vi "Data Logger.vi"() -> ()   [LabVIEW 2020]
uses:
  epl-vi-lib/Utility VIs/Buttons/KCheckmarkBoolean 2.ctl
  Typedefs/DL-Channel Spec.ctl
  <vilib>/DAQmx/read.llb/DAQmx Read (Analog 1D Wfm NChan NSamp).vi
  Typedefs/DL-Globals.vi
  <vilib>/DAQmx/miscellaneous.llb/DAQmx Fill In Error Info.vi
  <vilib>/sound2/lvsound2.llb/Sound File Write (DBL).vi
  <resource>/objmgr/daqmx.rc
panel:
  in  "Trigger":enum16{"Internal", "External"}(ring)
  in  ".wav file":T1 caption="Save as .wav file"
  in  "Duration (s)":dbl=1.0 min=1.0
  in  "Device":u16(ring) items=["PXI1Slot4"]
  in  "Filestem":string
  in  "Folder":path
  in  "Sampling rate (Hz)":dbl=1000.0 min=1000.0 max=200000.0
  in  "AI":T2
  out "Filename":string
  out "finished":errorcluster
  out "Graph":dbl[][](graph)
  in  "Start":bool
  in  "Stop":bool
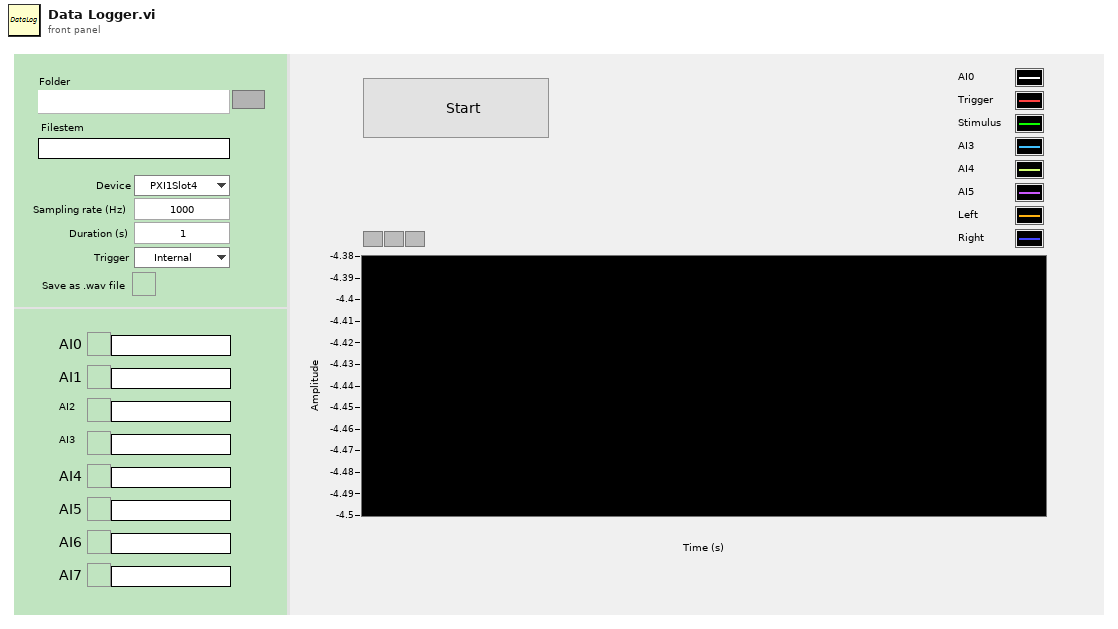
[diagram p1: front panel]
types:
  T1 = typedef "KCheckmarkBoolean 2.ctl" = bool
  T2 = cluster{"Ch0":cluster{"active":T1, "name":string}, "Ch1":cluster{"active":T1, "name":string}, "Ch2":cluster{"active":T1, "name":string}, "Ch3":cluster{"active":T1, "name":string}, "Ch4":cluster{"active":T1, "name":string}, "Ch5":cluster{"active":T1, "name":string}, "Ch6":cluster{"active":T1, "name":string}, "Ch7":cluster{"active":T1, "name":string}}
  T3 = typedef "DL-IPC.ctl" = cluster{"Acquire":refnum<queue>, "Analysis":refnum<queue>, "Data":refnum<queue>}
  T4 = typedef "DL-Channel Spec.ctl" = cluster{"active":bool, "name":string}
  T5 = enum8{"Enabled", "Disabled", "Disabled and Grayed Out"}
  T6 = typedef "DL-Configuration.ctl" = cluster{"Folder":path, "Filestem":string, "Device":string, "Fs (Hz)":dbl, "T (s)":dbl, "AI":T4[], "frame size (s)":dbl, ".wav file":bool, "Trigger":enum16{"Internal", "External"}, "remote":bool}
  T7 = typedef "Sound File Refnum.ctl" = refnum<file>
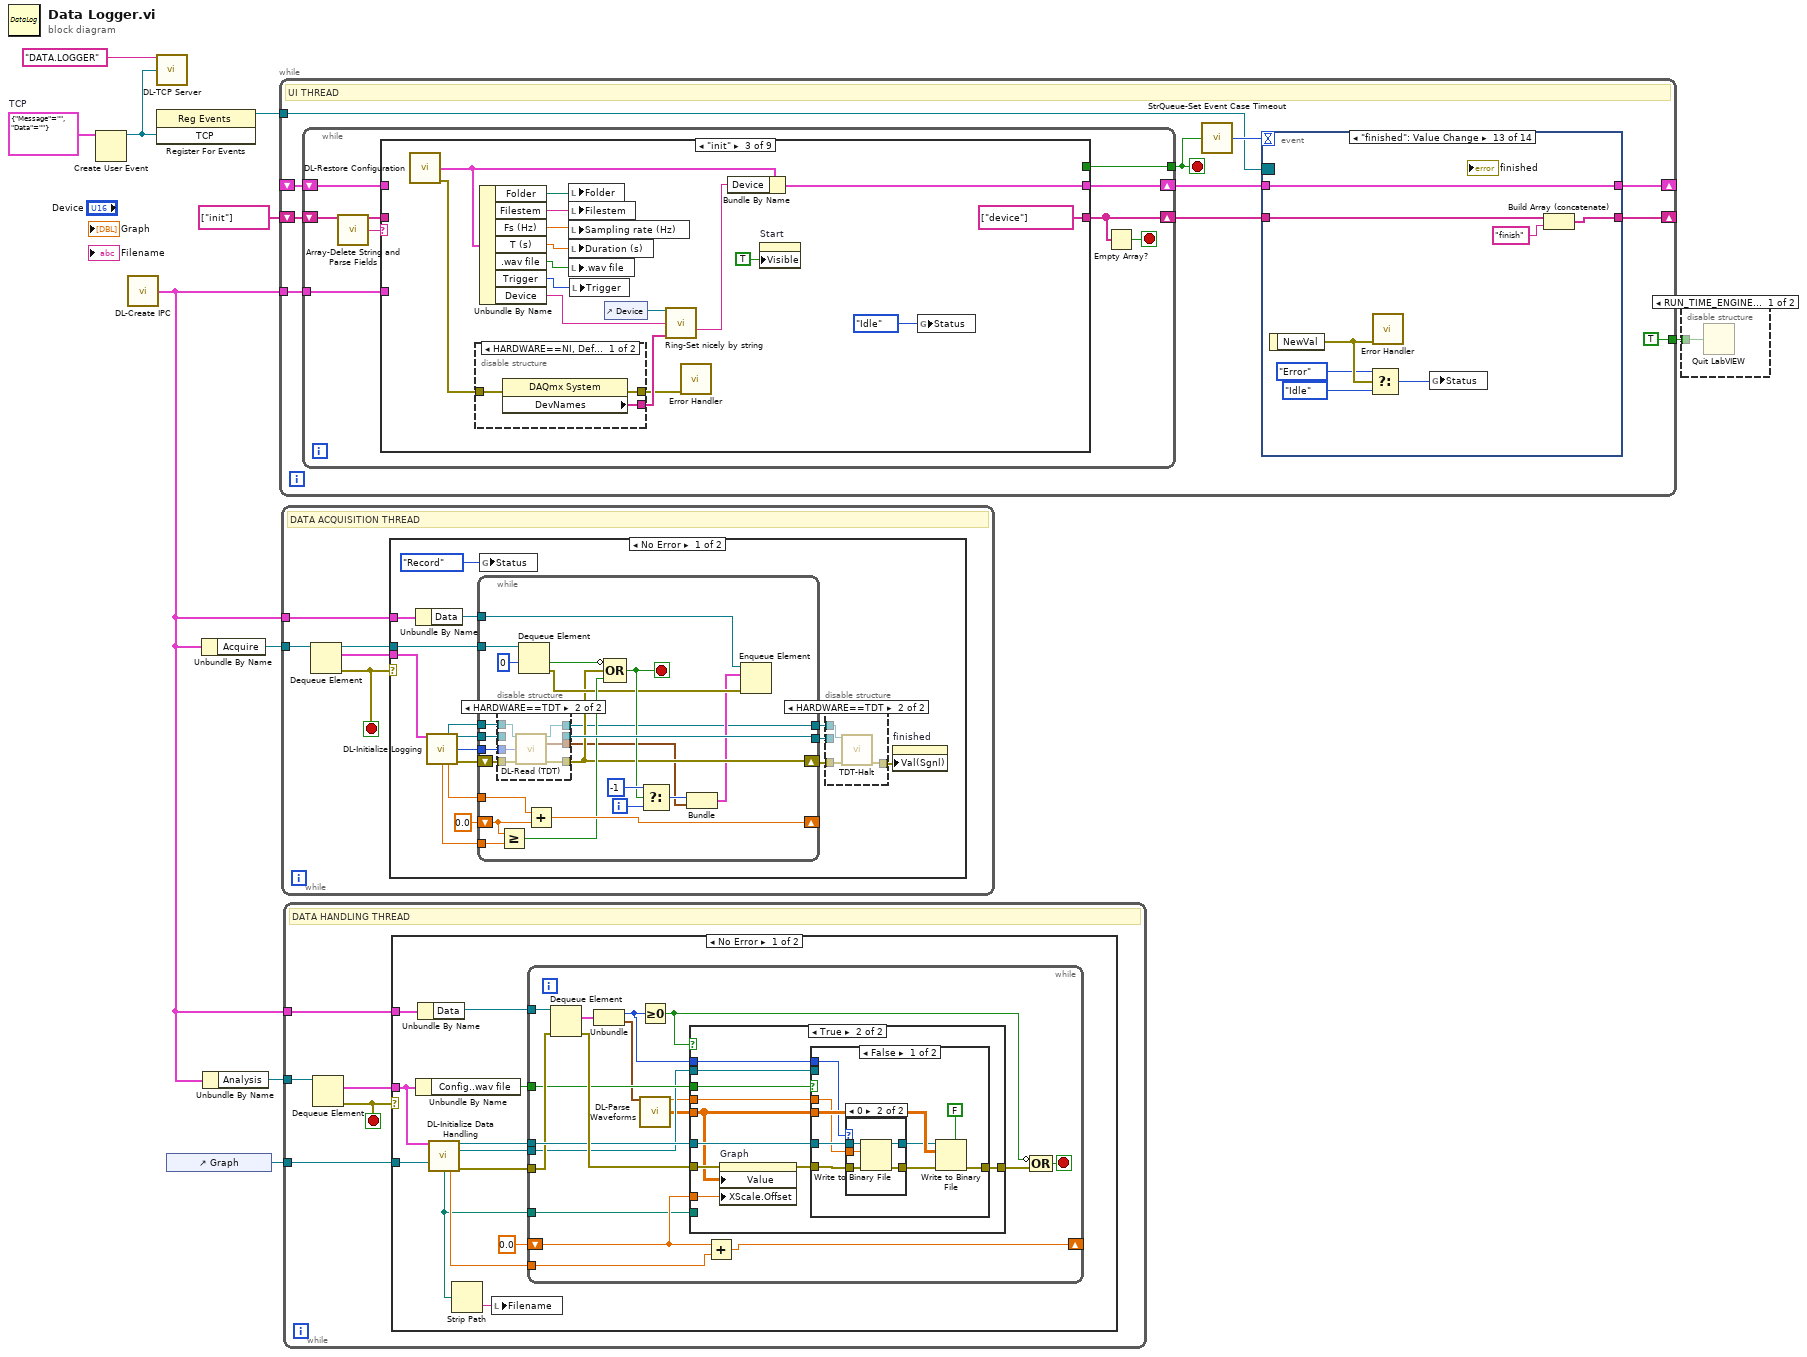
[diagram p0: block diagram]
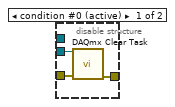
[diagram p2: hidden frame]
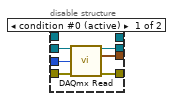
[diagram p3: hidden frame]
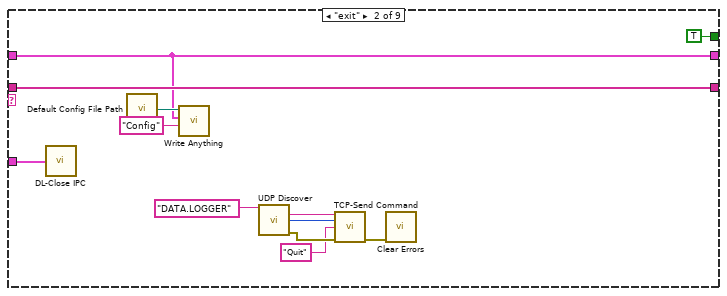
[diagram p6: hidden frame]
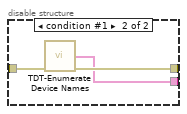
[diagram p7: hidden frame]
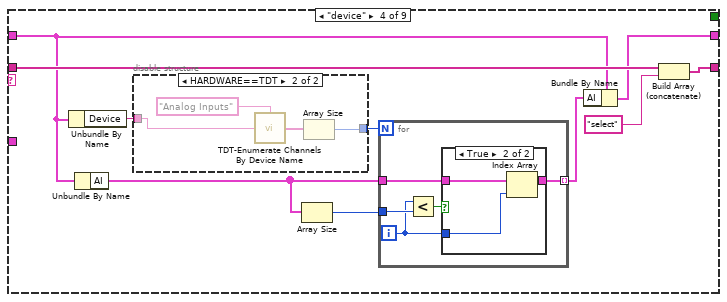
[diagram p8: hidden frame]
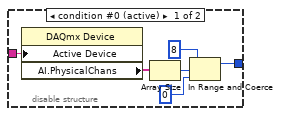
[diagram p9: hidden frame]
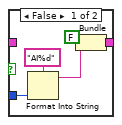
[diagram p10: hidden frame]
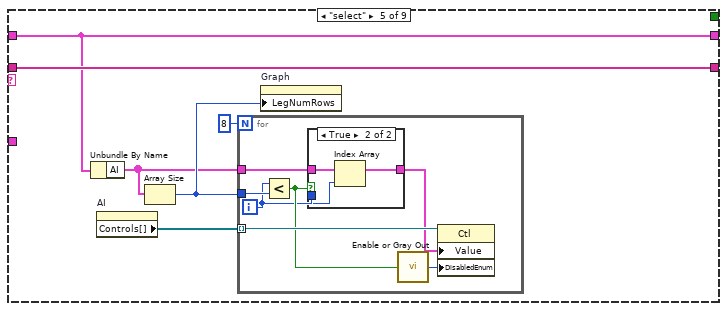
[diagram p11: hidden frame]
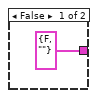
[diagram p12: hidden frame]
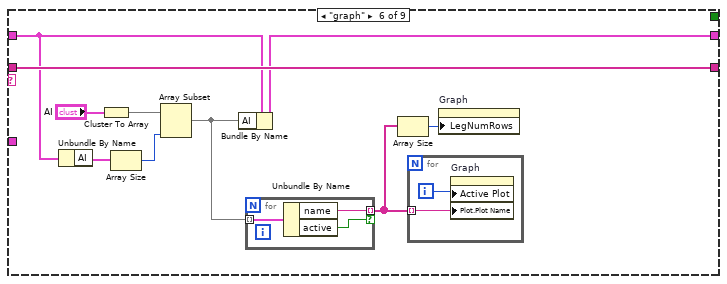
[diagram p13: hidden frame]
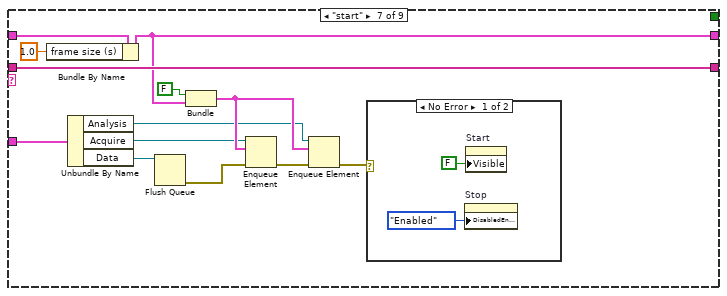
[diagram p14: hidden frame]
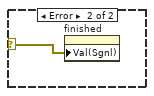
[diagram p15: hidden frame]
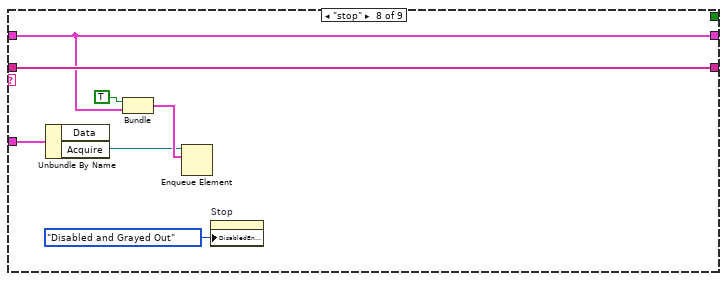
[diagram p16: hidden frame]
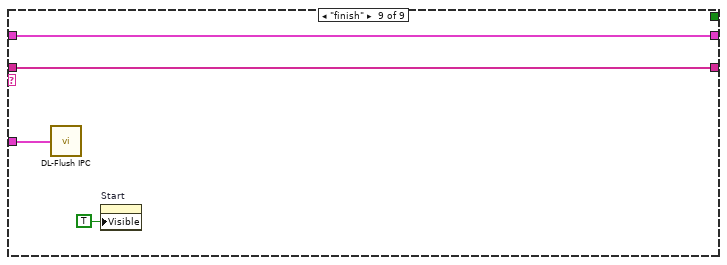
[diagram p17: hidden frame]
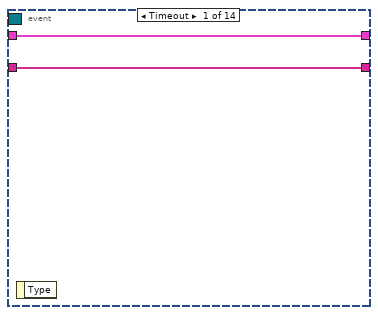
[diagram p18: hidden frame]
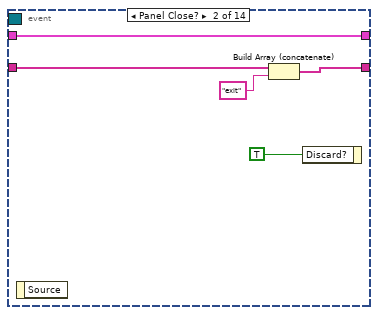
[diagram p19: hidden frame]
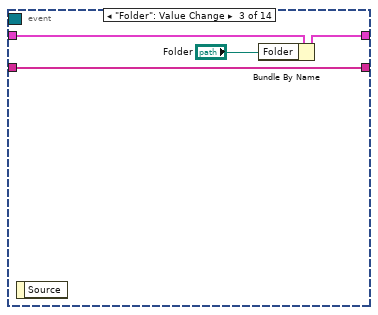
[diagram p20: hidden frame]
diagram:
  w1 = cluster{"Message":string, "Data":string} {"Message"="", "Data"=""}  # TCP
  n1 = Create User Event(user event datatype=w1) -> (user event=w2:refnum<user-event>)  [unwired: 1 in, 1 out]
  n2 = call "DL-Create IPC.vi"() -> ("IPC"=w8:T3)  [unwired: 15 in]
  n3 = call "DL-TCP Server.vi"("callsign"="DATA.LOGGER", "TCP Event"=w2) -> ()  [unwired: 14 in]
  n4 = register-events(w2) -> (reference out=w3:refnum<event-registration>)  [unwired: 2 in, 1 out]
  n5 = control-ref of="Graph"() -> (w7:refnum<vi>)
  n6 = Unbundle By Name(w8) -> ("Acquire"=w10:refnum<queue>)
  n7 = Unbundle By Name(w8) -> ("Analysis"=w9:refnum<queue>)
  n8 = while {
    shift-right: [w19] -> _
    shift-left: _ -> [w18]
    tunnel: w8 -> [w21]
    tunnel: [TRUE] -> w6
    shift-right: [w16] -> _
    shift-left: string[] ["init"] -> [w12]
    tunnel: w3 -> [w11]
    stop <- w13 stop-if-true
    # "UI THREAD"
    n9 = while {
      shift-right: [w30] -> w17
      shift-left: w12 -> [w27]
      tunnel: [w28] -> w13
      tunnel: w21 -> [w24]
      shift-right: [w23] -> w20
      shift-left: w18 -> [w22]
      stop <- w29 stop-if-true
      n10 = call "Array-Delete String and Parse Fields.vi"("Array in"=w27) -> ("Array out"=w26:string[], "Field 1"=w25:string)  [unwired: 10 in, 3 out]
      n11 = case shown="\"init\"" w25 {
        tunnel: w26 -> [w32 w44 _ w77 w106 w127 w145 w155 w159]
        tunnel: [w32 w44 string[] ["device"] ("Array out") w69 w106 w127 w145 w155 w159] -> w30
        tunnel: [_ TRUE _ _ _ _ _ _ _] -> w28
        tunnel: w24 -> [_ w43 _ _ _ _ w136 w151 w157]
        tunnel: [w31 w39 w50 w70 w101 w118 w134 w150 w158] -> w23
        tunnel: w22 -> [w31 w39 _ w71 w101 w119 w135 w150 w158]
        frame Default {
        }
        frame "exit" {
          n12 = call "DL-Close IPC.vi"("IPC"=w43) -> ()  [unwired: 14 in, 1 out]
          n13 = call "Default Config File Path.vi"() -> ("Default config file name"=w41:path)
          n14 = call "Write Anything.vi"("Section Name (Name of \"Anything\")"="Config" ("Section Name (Name of \"Anything\")"), "Anything"=w39, "Path (dialog)"=w41) -> ()  [unwired: 7 in, 2 out]
          n15 = call "UDP Discover.vi"("Name"="DATA.LOGGER" ("callsign")) -> ("Address"=w38:string, "Port"=w37:i32, "error out"=w36:errorcluster)  [unwired: 10 in, 2 out]
          n16 = call "TCP-Send Command.vi"("PXI Address"=w38, "Port"=w37, "Command"="Quit", "error in (no error)"=w36) -> ("error out"=w33:errorcluster)  [unwired: 11 in]
          n17 = call <vilib>:"Clear Errors.vi"("error in (no error)"=w33) -> ()  [unwired: 5 in, 2 out]
        }
        frame "init" {
          n18 = call "DL-Restore Configuration.vi"() -> ("Config"=w51:T6, "error out"=w48:errorcluster)  [unwired: 14 in]
          n19 = disable-structure shown="HARDWARE==NI, Default" {
            disable-tunnel: w48 -> [w63 w67]
            disable-tunnel: [w62 w65] -> w47
            disable-tunnel: [w64 w66] -> w46
            frame condition #0 (active) {
              n20 = property class="DAQmx System"(error in=w63) -> (error out=w64:errorcluster, "DevNames"=w62:tag[])  [unwired: 1 in, 1 out]
            }
            frame condition #1 {
              n21 = call "TDT-Enumerate Device Names.vi"("error in (no error)"=w67) -> ("Device names"=w65:string[], "error out"=w66:errorcluster)  [unwired: 13 in]
            }
          }
          n22 = Unbundle By Name(w51) -> ("Folder"=w52:path, "Filestem"=w53:string, "Fs (Hz)"=w54:dbl, "T (s)"=w57:dbl, ".wav file"=w59:bool, "Trigger"=w60:enum16{"Internal", "External"}, "Device"=w56:string)
          n23 = local write "Folder"(w52) -> ()
          n24 = local write "Filestem"(w53) -> ()
          n25 = local write "Sampling rate (Hz)"(w54) -> ()
          n26 = local write "Duration (s)"(w57) -> ()
          n27 = local write ".wav file"(w59) -> ()
          n28 = local write "Trigger"(w60) -> ()
          n29 = control-ref of="Device"() -> (w55:refnum<vi>)
          n30 = call "Ring-Set nicely by string.vi"("Ring in"=w55, "Device"=w56, "Strings []"=w47) -> ("Selection"=w61:string)  [unwired: 8 in, 4 out]
          n31 = call "Error Handler.vi"("error in (no error)"=w46) -> ()  [unwired: 12 in, 3 out]
          n32 = Bundle By Name(cluster=w51, "Device"=w61) -> (w50:T6)
          n33 = property on="Start" class="Bool"("Visible"=TRUE) -> ()  [unwired: 2 in, 2 out]
          n34 = global write "DL-Globals.vi" "Status"(enum16{"Idle", "Record", "Error"}."Idle" ("Status")) -> ()
        }
        frame "device" {
          n35 = Unbundle By Name(w71) -> ("Device"=w72:string)
          n36 = Unbundle By Name(w71) -> ("AI"=w73:T4[])
          n37 = disable-structure shown="HARDWARE==TDT" {
            disable-tunnel: [w83 w85] -> w76
            disable-tunnel: w72 -> [w80 w87]
            frame condition #0 (active) {
              n38 = property class="DAQmx Device"("Active Device"=w80) -> ("AI.PhysicalChans"=w81:tag[])  [unwired: 2 in, 2 out]
              n39 = Array Size(array=w81) -> (size(s)=w82:i32)
              n40 = In Range and Coerce(upper limit=8, x=w82, lower limit=0) -> (coerced(x)=w83:i32)  [unwired: 1 out]
            }
            frame condition #1 {
              n41 = call "TDT-Enumerate Channels By Device Name.vi"("Type"="Analog Inputs", "Device"=w87) -> ("IO Channels"=w86:string[])  [unwired: 13 in]
              n42 = Array Size(array=w86) -> (size(s)=w85:i32)
            }
          }
          n43 = Array Size(array=w73) -> (size(s)=w74:i32)
          n44 = for {
            N: w76 -> [_]
            tunnel: w73 -> [w91]
            tunnel: w74 -> [w92]
            tunnel: [w89] -> w75 mode=indexing
            i -> [w88]
            n45 = Less?(x=w88, y=w92) -> (x < y?=w90:bool)
            n46 = case shown="True" w90 {
              tunnel: w91 -> [_ w100]
              tunnel: [w96 w99] -> w89
              tunnel: w88 -> [w97 w98]
              frame False {
                n47 = Format Into String(format string="AI%d", w97) -> (resulting string=w93:string)  [unwired: 2 in, 1 out]
                n48 = Bundle(FALSE, w93) -> (w96:cluster{bool, string})  [unwired: 1 in]
              }
              frame True {
                n49 = Index Array(array=w100, index=w98) -> (element=w99:T4)
              }
            }
          }
          n50 = Bundle By Name(cluster=w71, "AI"=w75) -> (w70:T6)
          n51 = Build Array (concatenate)(w77, "select") -> (w69:string[])
        }
        frame "select" {
          n52 = Unbundle By Name(w101) -> ("AI"=w103:T4[])
          n53 = property on="AI" class="Clust (strict)"() -> ("Controls[]"=w104:refnum<vi>[])  [unwired: 2 in, 2 out]
          n54 = Array Size(array=w103) -> (size(s)=w105:i32)
          n55 = for {
            N: 8 -> [_]
            tunnel: w103 -> [w111]
            tunnel: w105 -> [w113]
            tunnel: w104 -> [w112] mode=indexing
            i -> [w107]
            n56 = Less?(x=w107, y=w113) -> (x < y?=w109:bool)
            n57 = case shown="True" w109 {
              tunnel: w111 -> [_ w117]
              tunnel: [T4 {"active"=FALSE, "name"=""} ("Channel") w115] -> w108
              tunnel: w107 -> [_ w116]
              frame False {
              }
              frame True {
                n58 = Index Array(array=w117, index=w116) -> (element=w115:T4)
              }
            }
            n59 = call "Enable or Gray Out.vi"("Boolean"=w109) -> ("Disabled"=w110:T5)
            n60 = property class="Ctl"(reference=w112, "Value"=w108, "DisabledEnum"=w110) -> ()  [unwired: 1 in, 2 out]
          }
          n61 = property on="Graph" class="WFGraph (strict)"("LegNumRows"=w105) -> ()  [unwired: 2 in, 2 out]
        }
        frame "graph" {
          n62 = Unbundle By Name(w119) -> ("AI"=w122:T4[])
          n63 = Cluster To Array(cluster="AI") -> (array=w121:cluster{"active":T1, "name":string}[])
          n64 = Array Size(array=w122) -> (size(s)=w123:i32)
          n65 = Array Subset(array=w121, length=w123) -> (w124:cluster{"active":T1, "name":string}[])  [unwired: 1 in]
          n66 = Bundle By Name(cluster=w119, "AI"=w124) -> (w118:T6)
          n67 = for {
            tunnel: w124 -> [w130] mode=indexing
            tunnel: [w129] -> w126 mode=indexing if=w128
            n68 = Unbundle By Name(w130) -> ("name"=w129:string, "active"=w128:T1)
          }
          n69 = Array Size(array=w126) -> (size(s)=w125:i32)
          n70 = for {
            tunnel: w126 -> [w131] mode=indexing
            i -> [w132]
            n71 = property on="Graph" class="WFGraph (strict)"("Active Plot"=w132, "Plot.Plot Name"=w131) -> ()  [unwired: 2 in, 2 out]
          }
          n72 = property on="Graph" class="WFGraph (strict)"("LegNumRows"=w125) -> ()  [unwired: 2 in, 2 out]
        }
        frame "start" {
          n73 = Bundle By Name(cluster=w135, "frame size (s)"=1.0) -> (w134:T6)
          n74 = Unbundle By Name(w136) -> ("Analysis"=w139:refnum<queue>, "Acquire"=w138:refnum<queue>, "Data"=w143:refnum<queue>)
          n75 = Flush Queue(queue=w143) -> (error out=w144:errorcluster)  [unwired: 1 in, 2 out]
          n76 = Bundle(FALSE, "Config"=w134) -> (w141:cluster{bool, "Config":T6})  [unwired: 1 in]
          n77 = Enqueue Element(queue=w138, element=w141, error in (no error)=w144) -> (error out=w140:errorcluster)  [unwired: 1 in, 2 out]
          n78 = Enqueue Element(queue=w139, element=w141, error in (no error)=w140) -> (error out=w142:errorcluster)  [unwired: 1 in, 2 out]
          n79 = case shown="No Error" w142 {
            selector: w142 -> [_ w148]
            frame No Error {
              n80 = property on="Stop" class="Bool"("DisabledEnum"=T5."Enabled" ("Disabled")) -> ()  [unwired: 2 in, 2 out]
              n81 = property on="Start" class="Bool"("Visible"=FALSE) -> ()  [unwired: 2 in, 2 out]
            }
            frame Error {
              n82 = property on="finished" class="Clust (strict)"("Val(Sgnl)"=w148) -> ()  [unwired: 2 in, 2 out]
            }
          }
        }
        frame "stop" {
          n83 = Unbundle By Name(w151) -> ("Acquire"=w153:refnum<queue>)  [unwired: 1 out]
          n84 = Bundle(TRUE, "Config"=w150) -> (w154:cluster{bool, "Config":T6})  [unwired: 1 in]
          n85 = Enqueue Element(queue=w153, element=w154) -> ()  [unwired: 2 in, 3 out]
          n86 = property on="Stop" class="Bool"("DisabledEnum"=T5."Disabled and Grayed Out" ("Disabled")) -> ()  [unwired: 2 in, 2 out]
        }
        frame "finish" {
          n87 = call "DL-Flush IPC.vi"("IPC"=w157) -> ()  [unwired: 14 in, 1 out]
          n88 = property on="Start" class="Bool"("Visible"=TRUE) -> ()  [unwired: 2 in, 2 out]
        }
      }
      n89 = Empty Array?(array=w30) -> (empty?=w29:bool)
    }
    n90 = call "StrQueue-Set Event Case Timeout.vi"("Quit"=w13) -> ("timeout"=w14:i32)  [unwired: 14 in]
    n91 = event shown="[12] \"finished\": Value Change" {
      selector: w11 -> [_ _ _ _ _ _ _ _ _ _ _ _ _ _]
      dyn-events: _ -> [_ _ _ _ _ _ _ _ _ _ _ _ _ _]
      timeout: w14 -> [_ _ _ _ _ _ _ _ _ _ _ _ _ _]
      tunnel: [w161 w165 w169 w173 w177 w181 w185 w189 w195 w200 w202 w210 w218 w223] -> w19
      tunnel: w20 -> [w161 w165 w170 w174 w178 w182 w186 w190 w196 w200 w206 w210 w218 w225]
      tunnel: w17 -> [w160 w164 w167 w171 w175 w179 w183 w187 w193 w199 w205 w209 w217 w226]
      tunnel: [w160 w163 w167 w171 w175 w179 w183 w187 w192 w198 w204 w208 w216 w220] -> w16
      event Timeout {
        n92 = event-data() -> ()  [unwired: 1 in, 1 out]
      }
      event Panel Close? {
        n93 = event-data() -> ()  [unwired: 1 in, 1 out]
        n94 = Build Array (concatenate)(w164, "exit") -> (w163:string[])
        n95 = event-data("Discard?"=TRUE) -> ()  [unwired: 1 in, 1 out]
      }
      event "Folder": Value Change {
        n96 = event-data() -> ()  [unwired: 1 in, 1 out]
        n97 = Bundle By Name(cluster=w170, "Folder"="Folder") -> (w169:T6)
      }
      event "Filestem": Value Change {
        n98 = event-data() -> ()  [unwired: 1 in, 1 out]
        n99 = Bundle By Name(cluster=w174, "Filestem"="Filestem") -> (w173:T6)
      }
      event "Sampling rate (Hz)": Value Change {
        n100 = event-data() -> ()  [unwired: 1 in, 1 out]
        n101 = Bundle By Name(cluster=w178, "Fs (Hz)"="Sampling rate (Hz)") -> (w177:T6)
      }
      event "Duration (s)": Value Change {
        n102 = event-data() -> ()  [unwired: 1 in, 1 out]
        n103 = Bundle By Name(cluster=w182, "T (s)"="Duration (s)") -> (w181:T6)
      }
      event "Trigger": Value Change {
        n104 = event-data() -> ()  [unwired: 1 in, 1 out]
        n105 = Bundle By Name(cluster=w186, "Trigger"="Trigger") -> (w185:T6)
      }
      event Value Change {
        n106 = event-data() -> ()  [unwired: 1 in, 1 out]
        n107 = Bundle By Name(cluster=w190, ".wav file"=".wav file") -> (w189:T6)
      }
      event "Device": Value Change {
        n108 = event-data() -> ()  [unwired: 1 in, 1 out]
        n109 = property on="Device" class="Ring (strict)"() -> ("RingText.Text"=w194:string)  [unwired: 2 in, 2 out]
        n110 = Bundle By Name(cluster=w196, "Device"=w194) -> (w195:T6)
        n111 = Build Array (concatenate)(w193, "device") -> (w192:string[])
      }
      event "AI": Value Change {
        n112 = event-data() -> ()  [unwired: 1 in, 1 out]
        n113 = Build Array (concatenate)(w199, "graph") -> (w198:string[])
      }
      event "Start": Value Change {
        n114 = event-data() -> ()  [unwired: 1 in, 1 out]
        n115 = Bundle By Name(cluster=w206, "remote"=FALSE) -> (w202:T6)
        n116 = Build Array (concatenate)(w205, "start") -> (w204:string[])
      }
      event "Stop": Value Change {
        n117 = event-data() -> ()  [unwired: 1 in, 1 out]
        n118 = Build Array (concatenate)(w209, "stop") -> (w208:string[])
      }
      event "finished": Value Change {
        n119 = event-data() -> ("NewVal"=w214:errorcluster)  [unwired: 1 in]
        n120 = Select(t=enum16{"Idle", "Record", "Error"}."Error" ("Status"), s=w214, f=enum16{"Idle", "Record", "Error"}."Idle" ("Status")) -> (s? t:f=w211:enum16{"Idle", "Record", "Error"})
        n121 = call "Error Handler.vi"("error in (no error)"=w214) -> ()  [unwired: 12 in, 3 out]
        n122 = global write "DL-Globals.vi" "Status"(w211) -> ()
        n123 = Build Array (concatenate)(w217, "finish") -> (w216:string[])
      }
      event User Event {
        n124 = event-data() -> ("Message"=w224:string, "Data"=w222:string)  [unwired: 1 in]
        n125 = String To Path(string=w222) -> (path=w221:path)
        n126 = case shown="\"Record\"" w224 {
          tunnel: w225 -> [w227 w235 w236]
          tunnel: [w227 w233 w236] -> w223
          tunnel: w221 -> [_ w234 _]
          tunnel: [_ w231 w237] -> w219
          frame Default {
          }
          frame "Record" {
            n127 = Strip Path(path=w234) -> (stripped path=w229:path)  [unwired: 1 out]
            n128 = call <vilib>:"Get File Extension.vi"("file"=w234) -> ("filename without extension"=w230:string)  [unwired: 6 in, 4 out]
            n129 = local write "Folder"(w229) -> ()
            n130 = local write "Filestem"(w230) -> ()
            n131 = Bundle By Name(cluster=w235, "remote"=TRUE, "Folder"=w229, "Filestem"=w230) -> (w233:T6)
            n132 = Build Array("start") -> (w231:string[])
          }
          frame "Stop" {
            n133 = Build Array("stop") -> (w237:string[])
          }
        }
        n134 = Build Array (concatenate)(w226, w219) -> (w220:string[])
      }
    }
  }
  n135 = while {
    tunnel: w10 -> [w243]
    tunnel: w8 -> [w240]
    stop <- w242 stop-if-true
    # "DATA ACQUISITION THREAD"
    n136 = Dequeue Element(queue=w243) -> (queue out=w241:refnum<queue>, element=w239:cluster{"Stop":bool, "Config":T6}, error out=w242:errorcluster)  [unwired: 2 in, 1 out]
    n137 = case shown="No Error" w242 {
      tunnel: w241 -> [w257 _]
      tunnel: w240 -> [w255 _]
      tunnel: w239 -> [w247 _]
      frame No Error {
        n138 = Unbundle By Name(w255) -> ("Data"=w254:refnum<queue>)
        n139 = call "DL-Initialize Logging.vi"("Configuration"=w247) -> ("RPcoX"=w246:refnum<k7>, "task"=w259:refnum<k21>, "Npts"=w256:i32, "Config.T (s)"=w249:dbl, "Config.frame size (s)"=w248:dbl, "error out"=w258:errorcluster)  [unwired: 9 in]
        n140 = while {
          tunnel: w259 -> [w287]
          tunnel: w257 -> [w288]
          tunnel: w256 -> [w285]
          tunnel: w254 -> [w282]
          tunnel: [w281] -> w251
          shift-right: [w278] -> _
          shift-left: 0.0 -> [w280]
          tunnel: w249 -> [w279]
          tunnel: w248 -> [w277]
          shift-right: [w270] -> w253
          shift-left: w258 -> [w286]
          tunnel: [w267] -> w245
          tunnel: w246 -> [w266]
          i -> [w275]
          stop <- w272 stop-if-true
          n141 = disable-structure shown="HARDWARE==TDT" {
            disable-tunnel: w287 -> [w294 _]
            disable-tunnel: w286 -> [w293 w297]
            disable-tunnel: w285 -> [w292 w296]
            disable-tunnel: [w291 _] -> w281
            disable-tunnel: [w290 w298] -> w270
            disable-tunnel: [w289 w295] -> w268
            disable-tunnel: [_ w300] -> w267
            disable-tunnel: w266 -> [_ w299]
            frame condition #0 (active) {
              n142 = call-poly <vilib>:"DAQmx Read.vi"("task/channels in"=w294, "number of samples per channel"=w292, "error in"=w293) -> ("task out"=w291:refnum<k21>, "data"=w289:waveform(dbl)[], "error out"=w290:errorcluster)  [unwired: 10 in]
            }
            frame condition #1 {
              n143 = call "DL-Read (TDT).vi"("RPcoX in"=w299, "Npts"=w296, "error in (no error)"=w297) -> ("RPcoX out"=w300:refnum<k7>, "data"=w295:waveform(dbl)[], "error out"=w298:errorcluster)  [unwired: 10 in]
            }
          }
          n144 = Greater Or Equal?(x=w280, y=w279) -> (x >= y?=w276:bool)
          n145 = Dequeue Element(queue=w288, timeout in ms (-1)=0) -> (timed out?=w283:bool, error out=w271:errorcluster)  [unwired: 1 in, 2 out]
          n146 = Add(x=w277, y=w280) -> (x+y=w278:dbl)
          n147 = Compound Arithmetic op=OR(invert w283, w270, w276) -> (w272:bool)
          n148 = Select(t=-1, s=w272, f=w275) -> (s? t:f=w273:i32)
          n149 = Bundle("t"=w273, "data"=w268) -> (w269:cluster{"t":i32, "data":waveform(dbl)[]})  [unwired: 1 in]
          n150 = Enqueue Element(queue=w282, element=w269, error in (no error)=w271) -> ()  [unwired: 1 in, 3 out]
        }
        n151 = global write "DL-Globals.vi" "Status"(enum16{"Idle", "Record", "Error"}."Record" ("Status")) -> ()
        n152 = disable-structure shown="HARDWARE==TDT" {
          disable-tunnel: w253 -> [w262 w264]
          disable-tunnel: [w261 w265] -> w252
          disable-tunnel: w251 -> [w260 _]
          disable-tunnel: w245 -> [_ w263]
          frame condition #0 (active) {
            n153 = call <vilib>:"DAQmx Clear Task.vi"("task in"=w260, "error in"=w262) -> ("error out"=w261:errorcluster)  [unwired: 13 in]
          }
          frame condition #1 {
            n154 = call "TDT-Halt.vi"("RPcoX"=w263, "error in (no error)"=w264) -> ("error out"=w265:errorcluster)  [unwired: 13 in]
          }
        }
        n155 = property on="finished" class="Clust (strict)"("Val(Sgnl)"=w252) -> ()  [unwired: 2 in, 2 out]
      }
      frame Error {
      }
    }
  }
  n156 = while {
    tunnel: w9 -> [w305]
    tunnel: w8 -> [w302]
    tunnel: w7 -> [w301]
    stop <- w304 stop-if-true
    # "DATA HANDLING THREAD"
    n157 = Dequeue Element(queue=w305) -> (element=w303:cluster{"Stop":bool, "Config":T6}, error out=w304:errorcluster)  [unwired: 2 in, 2 out]
    n158 = case shown="No Error" w304 {
      tunnel: w303 -> [w310 _]
      tunnel: w302 -> [w316 _]
      tunnel: w301 -> [w314 _]
      frame No Error {
        n159 = Unbundle By Name(w310) -> ("Config..wav file"=w309:bool)
        n160 = Unbundle By Name(w316) -> ("Data"=w315:refnum<queue>)
        n161 = call "DL-Initialize Data Handling.vi"("Configuration"=w310, "Graph Ref"=w314) -> ("file"=w311:refnum<file>, ".wav"=w308:T7, "path"=w306:path, "frame size (s)"=w312:dbl, "error out"=w317:errorcluster)  [unwired: 9 in]
        n162 = Strip Path(path=w306) -> (name=w307:string)  [unwired: 1 out]
        n163 = local write "Filename"(w307) -> ()
        n164 = while {
          tunnel: w317 -> [w325]
          tunnel: w315 -> [w334]
          shift-right: [w328] -> _
          shift-left: 0.0 -> [w329]
          tunnel: w312 -> [w327]
          tunnel: w311 -> [w326]
          tunnel: w309 -> [w324]
          tunnel: w308 -> [w323]
          tunnel: w306 -> [w322]
          stop <- w335 stop-if-true
          n165 = Dequeue Element(queue=w334, error in (no error)=w325) -> (element=w333:cluster{"Num":i32, "data":waveform(dbl)[]}, error out=w332:errorcluster)  [unwired: 1 in, 2 out]
          n166 = Unbundle(w333) -> ("Num"=w318:i32, "data"=w321:waveform(dbl)[])
          n167 = Greater Or Equal To 0?(x=w318) -> (x >= 0?=w331:bool)
          n168 = call "DL-Parse Waveforms.vi"("Waveform array"=w321) -> ("timestamp"=w319:dbl, "2D Array"=w320:dbl[][])  [unwired: 13 in]
          n169 = case shown="True" w331 {
            tunnel: w332 -> [w343 w364]
            tunnel: w320 -> [_ w359]
            tunnel: [w338 w361] -> w330
            tunnel: w329 -> [w340 w363]
            tunnel: w326 -> [w344 w360]
            tunnel: w324 -> [w342 w358]
            tunnel: w323 -> [w341 w357]
            tunnel: w322 -> [w336 _]
            tunnel: w319 -> [_ w355]
            tunnel: w318 -> [_ w356]
            frame False {
              n170 = case shown="True" w342 {
                tunnel: w344 -> [w351 _]
                tunnel: w343 -> [w350 w353]
                tunnel: [w349 w352] -> w337
                tunnel: w341 -> [_ w354]
                frame False {
                  n171 = Close File(refnum=w351, error in=w350) -> (error out=w349:errorcluster)  [unwired: 1 out]
                }
                frame True {
                  n172 = call <vilib>:"Sound File Close.vi"("error in (no error)"=w353, "sound file refnum"=w354) -> ("error out"=w352:errorcluster)  [unwired: 9 in]
                }
              }
              n173 = Equal To 0?(x=w340) -> (x = 0?=w339:bool)
              n174 = case shown="True" w339 {
                tunnel: [w345 w348] -> w338
                tunnel: w337 -> [w345 w348]
                tunnel: [_ w347] -> _
                tunnel: w336 -> [_ w346]
                frame False {
                }
                frame True {
                  n175 = Delete(path (use dialog)=w346) -> (error out=w347:errorcluster)  [unwired: 4 in, 2 out]
                }
              }
            }
            frame True {
              n176 = property on="Graph" class="WFGraph (strict)"(error in=w364, "Value"=w359, "XScale.Offset"=w363) -> (error out=w362:errorcluster)  [unwired: 1 in, 1 out]
              n177 = case shown="False" w358 {
                tunnel: w362 -> [w370 w383]
                tunnel: [w373 w382] -> w361
                tunnel: w360 -> [w368 _]
                tunnel: w359 -> [w371 w385]
                tunnel: w357 -> [_ w381]
                tunnel: w356 -> [w365 _]
                tunnel: w355 -> [w366 _]
                frame False {
                  n178 = case shown="0" w365 {
                    tunnel: w370 -> [w374 w380]
                    tunnel: [w374 w379] -> w369
                    tunnel: w368 -> [w375 w378]
                    tunnel: [w375 w377] -> w367
                    tunnel: w366 -> [_ w376]
                    frame 1, Default {
                    }
                    frame 0 {
                      n179 = Write to Binary File(file (use dialog)=w378, data=w376, error in=w380) -> (refnum out=w377:refnum<file>, error out=w379:errorcluster)  [unwired: 3 in, 1 out]
                    }
                  }
                  n180 = Write to Binary File(file (use dialog)=w367, data=w371, error in=w369, 5:FALSE ("prepend array or string size? (T)")) -> (error out=w373:errorcluster)  [unwired: 2 in, 2 out]
                }
                frame True {
                  n181 = for {
                    tunnel: w385 -> [w387] mode=indexing
                    tunnel: [w386] -> w384 mode=indexing
                    n182 = Bundle By Name("Y"=w387) -> (w386:waveform(dbl))  [unwired: 1 in]
                  }
                  n183 = call-poly <vilib>:"Sound File Write.vi"("error in (no error)"=w383, "data"=w384, "sound file refnum"=w381) -> ("error out"=w382:errorcluster)  [unwired: 7 in, 1 out]
                }
              }
            }
          }
          n184 = Add(x=w329, y=w327) -> (x+y=w328:dbl)
          n185 = Compound Arithmetic op=OR(invert w331, w330) -> (w335:bool)
        }
      }
      frame Error {
      }
    }
  }
  n186 = disable-structure shown="RUN_TIME_ENGINE==True" {
    disable-tunnel: w6 -> [w388 _]
    frame condition #0 {
      n187 = Quit LabVIEW(quit? (T)=w388) -> ()
    }
    frame condition #1 (active) {
    }
  }
